vi "REF phase equals zero.vi"(10 "reset REF phi to zero":bool, 11 "Cluster out 3":T1) -> (3 "Cluster out 2":T1)   [LabVIEW 2013]
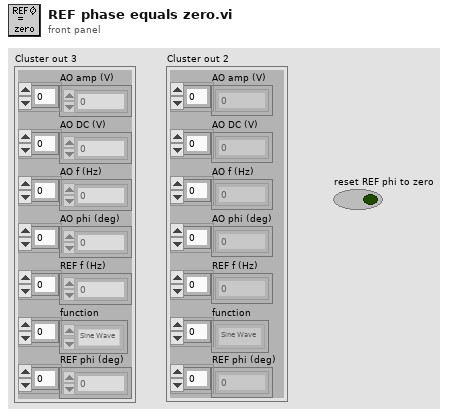
[diagram p1: front panel]
types:
  T1 = cluster{"AO amp (V)":dbl[], "AO DC (V)":dbl[], "AO f (Hz)":dbl[], "AO phi (deg)":dbl[], "REF f (Hz)":dbl[], "function":enum16{"Sine Wave", "Triangle Wave", "Square Wave", "Sawtooth Wave"}[], "REF phi (deg)":dbl[]}
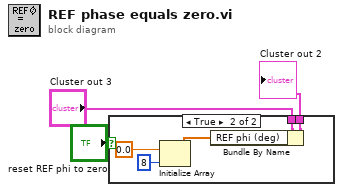
[diagram p0: block diagram]
diagram:
  n1 = case shown="True" "reset REF phi to zero" {
    tunnel: "Cluster out 3" -> [w4 w6]
    tunnel: [w4 w5] -> w2
    frame False {
    }
    frame True {
      n2 = Initialize Array(0.0, 8 ("dimension size")) -> (w7:dbl[])
      n3 = Bundle By Name(cluster=w6, "REF phi (deg)"=w7) -> (w5:T1)
    }
  }
  "Cluster out 2" <- w2
